vi "Get Border Index.vi"(4 "Y Dimension":i32, 6 "X Dimension":i32, 9 "Min Z":sgl, 11 "Border Vertex Array In":cluster{"X":sgl, "Y":sgl, "Z":sgl}[](array[cluster])) -> (1 "Polygens Index Array":u32[](array[numeric]), 2 "Wireframe Index Array":u32[](array[numeric]), 3 "Border Vertex Array Out":cluster{"X":sgl, "Y":sgl, "Z":sgl}[](array[cluster]))   [LabVIEW 2017, in "3D Mesh.lvclass"]
uses:
  <vilib>/Math Plots/3D Math Plots/3D Mesh/3D Mesh/3D Mesh.lvclass
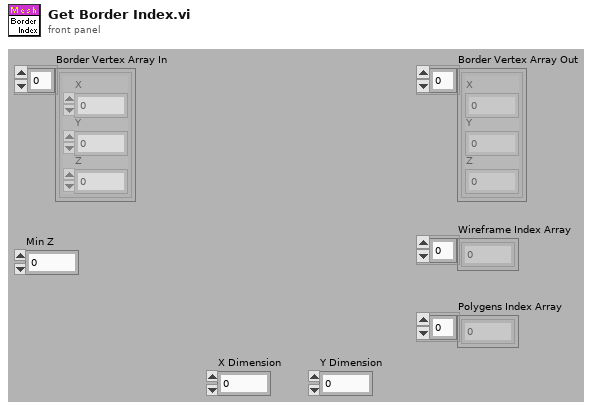
[diagram p1: front panel]
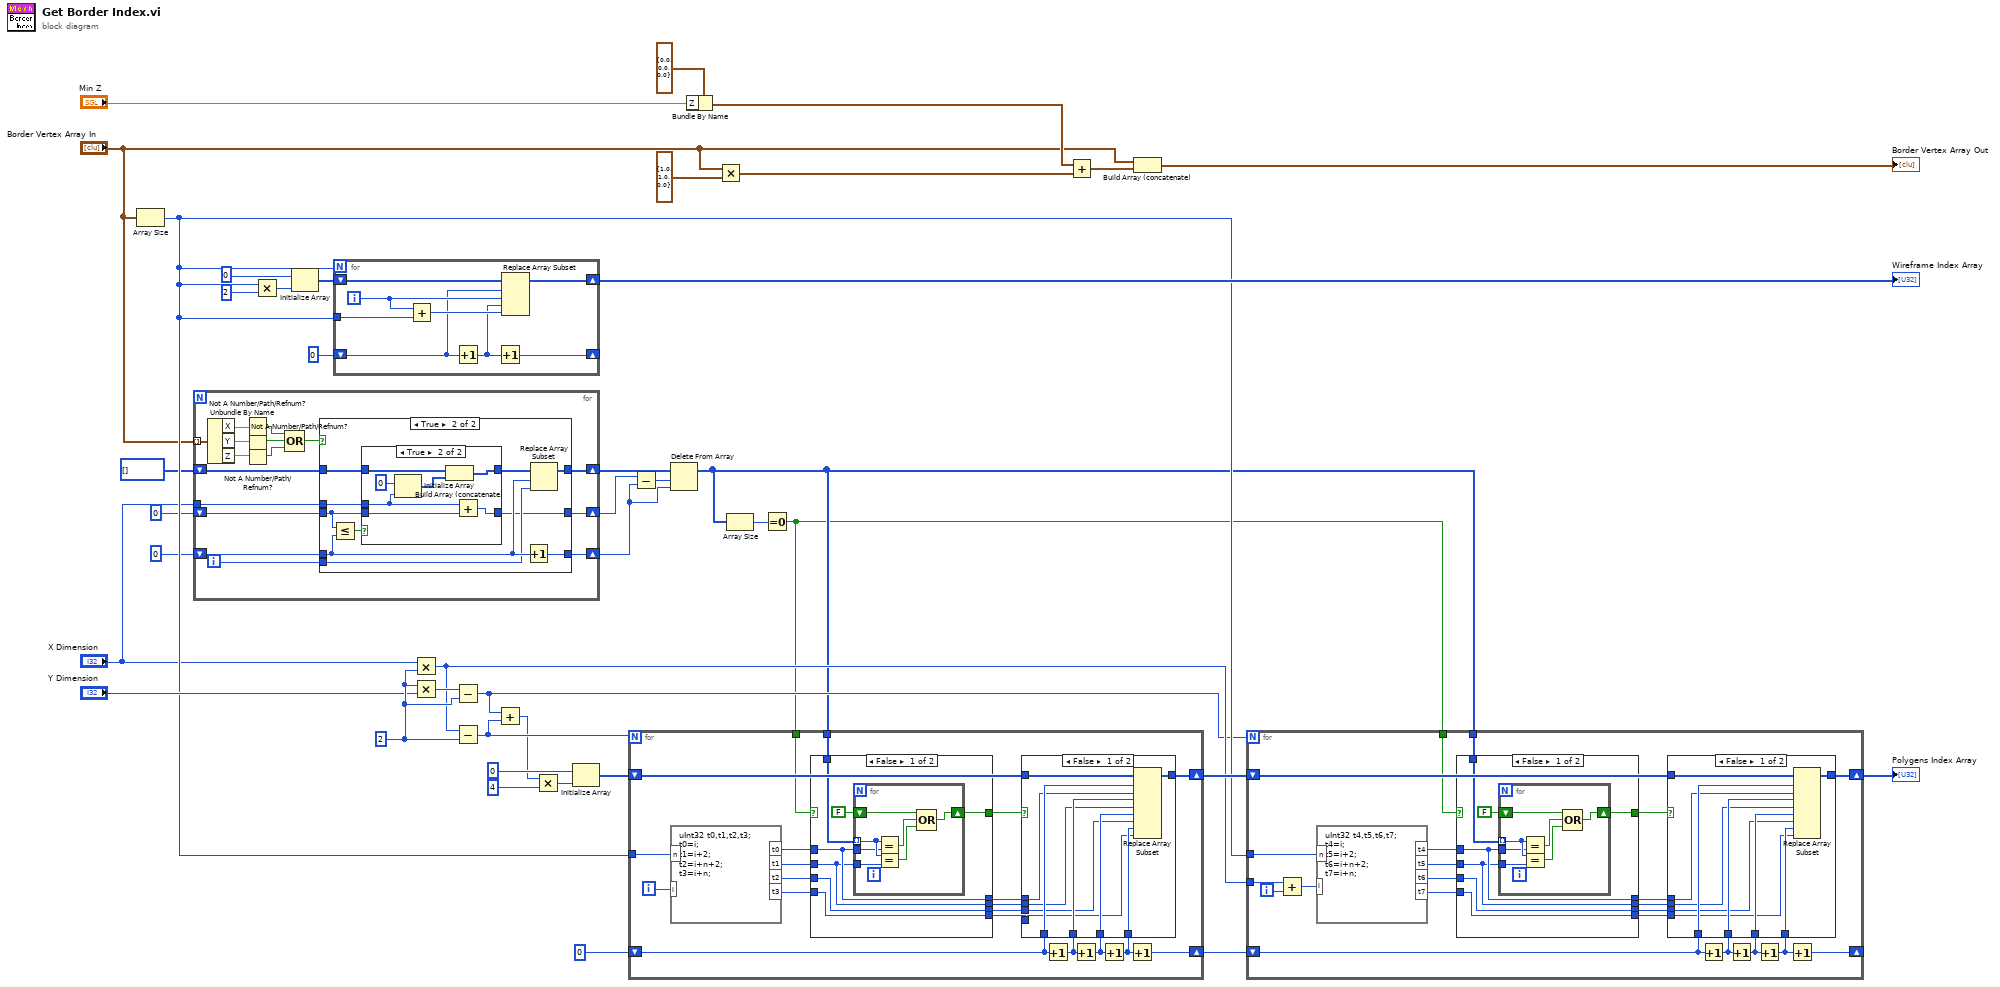
[diagram p0: block diagram]
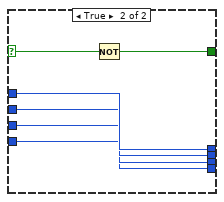
[diagram p5: hidden frame]
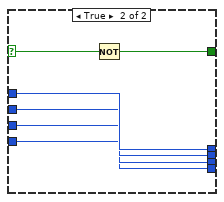
[diagram p7: hidden frame]
diagram:
  w33 = 2 ("y")
  n1 = Array Size(array="Border Vertex Array In") -> (size(s)=w24:i32)
  n2 = for {
    tunnel: "Border Vertex Array In" -> [w57] mode=indexing
    shift-right: [w46] -> w5
    shift-left: 0 -> [w43]
    shift-right: [w47] -> w4
    shift-left: 0 -> [w44]
    shift-right: [w48] -> w6
    shift-left: u32[] [] -> [w45]
    tunnel: "X Dimension" -> [w42]
    i -> [w49]
    n3 = Unbundle By Name(w57) -> ("X"=w56:sgl, "Y"=w55:sgl, "Z"=w54:sgl)
    n4 = Not A Number/Path/Refnum?(number/path/refnum=w56) -> (NaN/Path/Refnum?=w53:bool)
    n5 = Not A Number/Path/Refnum?(number/path/refnum=w55) -> (NaN/Path/Refnum?=w52:bool)
    n6 = Not A Number/Path/Refnum?(number/path/refnum=w54) -> (NaN/Path/Refnum?=w51:bool)
    n7 = Compound Arithmetic op=OR(w53, w52, w51) -> (w50:bool)
    n8 = case shown="True" w50 {
      tunnel: w45 -> [w60 w68]
      tunnel: [w60 w64] -> w48
      tunnel: w49 -> [_ w65]
      tunnel: w43 -> [w59 w66]
      tunnel: [w59 w70] -> w46
      tunnel: w44 -> [w58 w62]
      tunnel: [w58 w63] -> w47
      tunnel: w42 -> [_ w61]
      frame False {
      }
      frame True {
        n9 = Less Or Equal?(x=w62, y=w66) -> (x <= y?=w69:bool)
        n10 = case shown="True" w69 {
          tunnel: w68 -> [w72 w79]
          tunnel: [w72 w78] -> w67
          tunnel: [w71 w74] -> w63
          tunnel: w62 -> [w71 w75]
          tunnel: w61 -> [_ w73]
          frame False {
          }
          frame True {
            n11 = Initialize Array(u32 0, w73) -> (w76:u32[])
            n12 = Build Array (concatenate)(w79, w76) -> (w78:u32[])
            n13 = Add(x=w73, y=w75) -> (x+y=w74:i32)
          }
        }
        n14 = Increment(x=w66) -> (x+1=w70:i32)
        n15 = Replace Array Subset(array=w67, new element=w65, index=w66) -> (w64:u32[])
      }
    }
  }
  n16 = Multiply(x=w24, y=2) -> (x*y=w25:i32)
  n17 = Initialize Array(u32 0, w25) -> (w26:u32[])
  n18 = for {
    N: w24 -> [_]
    shift-right: [w86] -> w39
    shift-left: w26 -> [w87]
    tunnel: w24 -> [w85]
    shift-right: [w82] -> _
    shift-left: 0 ("y") -> [w81]
    i -> [w83]
    n19 = Add(x=w83, y=w85) -> (x+y=w84:i32)
    n20 = Increment(x=w81) -> (x+1=w80:i32)
    n21 = Increment(x=w80) -> (x+1=w82:i32)
    n22 = Replace Array Subset(array=w87, new element #1=w83, index #1=w81, new element #2=w84, index #2=w80) -> (w86:u32[])
  }
  "Wireframe Index Array" <- w39
  n23 = Multiply(x="X Dimension", y=w33) -> (x*y=w32:i32)
  n24 = Multiply(x=w33, y="Y Dimension") -> (x*y=w34:i32)
  n25 = Subtract(x=w34, y=w33) -> (x-y=w18:i32)
  n26 = Subtract(x=w32, y=w33) -> (x-y=w17:i32)
  n27 = Add(x=w18, y=w17) -> (x+y=w16:i32)
  n28 = Multiply(x=w16, y=4) -> (x*y=w20:i32)
  n29 = Initialize Array(u32 0, w20) -> (w15:u32[])
  n30 = Subtract(x=w4, y=w5) -> (x-y=w7:i32)
  n31 = Delete From Array(array=w6, length=w7, index=w5) -> (array with subset deleted=w2:u32[])  [unwired: 1 out]
  n32 = Bundle By Name(cluster=cluster{"X":sgl, "Y":sgl, "Z":sgl} {"X"=0.0, "Y"=0.0, "Z"=0.0} ("3D Point 2"), "Z"="Min Z") -> (w37:cluster{"X":sgl, "Y":sgl, "Z":sgl})
  n33 = Multiply(x="Border Vertex Array In", y=cluster{"X":sgl, "Y":sgl, "Z":sgl} {"X"=1.0, "Y"=1.0, "Z"=0.0} ("3D Point 2")) -> (x*y=w38:cluster{"X":sgl, "Y":sgl, "Z":sgl}[])
  n34 = Array Size(array=w2) -> (size(s)=w3:i32)
  n35 = Equal To 0?(x=w3) -> (x = 0?=w1:bool)
  n36 = for {
    N: w17 -> [_]
    shift-right: [w106] -> w35
    shift-left: w15 -> [w107]
    tunnel: w24 -> [w105]
    shift-right: [w103] -> w13
    shift-left: 0 ("y") -> [w102]
    tunnel: w1 -> [w98]
    tunnel: w2 -> [w97]
    i -> [w104]
    n37 = formula code="uInt32 t0,t1,t2,t3;\nt0=i;\nt1=i+2;\nt2=i+n+2;\nt3=i+n;"("n"=w105, "i"=w104) -> ("t0"=w96:u32, "t1"=w95:u32, "t2"=w94:u32, "t3"=w93:u32)
    n38 = case shown="False" w98 {
      selector: w98 -> [_ w134]
      tunnel: [w122 w138] -> w92
      tunnel: w96 -> [w122 w138]
      tunnel: [w121 w137] -> w91
      tunnel: w95 -> [w121 w137]
      tunnel: [w120 w136] -> w90
      tunnel: w94 -> [w120 w136]
      tunnel: [w119 w135] -> w89
      tunnel: w93 -> [w119 w135]
      tunnel: w97 -> [w125 _]
      tunnel: [w123 w133] -> w88
      frame False {
        n39 = for {
          tunnel: w125 -> [w132] mode=indexing
          tunnel: w122 -> [w131]
          tunnel: w121 -> [w126]
          shift-right: [w128] -> w123
          shift-left: FALSE -> [w127]
          n40 = Equal?(x=w132, y=w131) -> (x = y?=w130:bool)
          n41 = Equal?(x=w132, y=w126) -> (x = y?=w129:bool)
          n42 = Compound Arithmetic op=OR(w127, w130, w129) -> (w128:bool)
        }
      }
      frame True {
        n43 = Not(x=w134) -> (.not. x?=w133:bool)
      }
    }
    n44 = Increment(x=w102) -> (x+1=w101:i32)
    n45 = Increment(x=w101) -> (x+1=w100:i32)
    n46 = Increment(x=w100) -> (x+1=w99:i32)
    n47 = case shown="False" w88 {
      tunnel: w107 -> [w117 w118]
      tunnel: [w116 w118] -> w106
      tunnel: w102 -> [w115 _]
      tunnel: w101 -> [w114 _]
      tunnel: w100 -> [w113 _]
      tunnel: w99 -> [w112 _]
      tunnel: w92 -> [w111 _]
      tunnel: w91 -> [w110 _]
      tunnel: w90 -> [w109 _]
      tunnel: w89 -> [w108 _]
      frame False {
        n48 = Replace Array Subset(array=w117, new element #1=w111, index #1=w115, new element #2=w110, index #2=w114, new element #3=w109, index #3=w113, new element #4=w108, index #4=w112) -> (w116:u32[])
      }
      frame True {
      }
    }
    n49 = Increment(x=w99) -> (x+1=w103:i32)
  }
  n50 = Add(x=w37, y=w38) -> (x+y=w36:cluster{"X":sgl, "Y":sgl, "Z":sgl}[])
  n51 = Build Array (concatenate)("Border Vertex Array In", w36) -> (→"Border Vertex Array Out":cluster{"X":sgl, "Y":sgl, "Z":sgl}[])
  n52 = for {
    N: w18 -> [_]
    shift-right: [w155] -> w31
    shift-left: w35 -> [w156]
    tunnel: w24 -> [w160]
    tunnel: w32 -> [w159]
    shift-right: [w154] -> _
    shift-left: w13 -> [w153]
    tunnel: w2 -> [w149]
    tunnel: w1 -> [w148]
    i -> [w158]
    n53 = Add(x=w159, y=w158) -> (x+y=w157:i32)
    n54 = formula code="uInt32 t4,t5,t6,t7;\nt4=i;\nt5=i+2;\nt6=i+n+2;\nt7=i+n;"("n"=w160, "i"=w157) -> ("t4"=w147:u32, "t5"=w146:u32, "t6"=w145:u32, "t7"=w144:u32)
    n55 = case shown="False" w148 {
      selector: w148 -> [_ w187]
      tunnel: [w175 w191] -> w143
      tunnel: w147 -> [w175 w191]
      tunnel: [w174 w190] -> w142
      tunnel: w146 -> [w174 w190]
      tunnel: [w173 w189] -> w141
      tunnel: w145 -> [w173 w189]
      tunnel: [w172 w188] -> w140
      tunnel: w144 -> [w172 w188]
      tunnel: w149 -> [w178 _]
      tunnel: [w176 w186] -> w139
      frame False {
        n56 = for {
          tunnel: w178 -> [w185] mode=indexing
          tunnel: w175 -> [w184]
          tunnel: w174 -> [w179]
          shift-right: [w181] -> w176
          shift-left: FALSE -> [w180]
          n57 = Equal?(x=w185, y=w184) -> (x = y?=w183:bool)
          n58 = Equal?(x=w185, y=w179) -> (x = y?=w182:bool)
          n59 = Compound Arithmetic op=OR(w180, w183, w182) -> (w181:bool)
        }
      }
      frame True {
        n60 = Not(x=w187) -> (.not. x?=w186:bool)
      }
    }
    n61 = Increment(x=w153) -> (x+1=w152:i32)
    n62 = Increment(x=w152) -> (x+1=w151:i32)
    n63 = Increment(x=w151) -> (x+1=w150:i32)
    n64 = case shown="False" w139 {
      tunnel: w156 -> [w170 w171]
      tunnel: [w169 w171] -> w155
      tunnel: w153 -> [w168 _]
      tunnel: w152 -> [w167 _]
      tunnel: w151 -> [w166 _]
      tunnel: w150 -> [w165 _]
      tunnel: w143 -> [w164 _]
      tunnel: w142 -> [w163 _]
      tunnel: w141 -> [w162 _]
      tunnel: w140 -> [w161 _]
      frame False {
        n65 = Replace Array Subset(array=w170, new element #1=w164, index #1=w168, new element #2=w163, index #2=w167, new element #3=w162, index #3=w166, new element #4=w161, index #4=w165) -> (w169:u32[])
      }
      frame True {
      }
    }
    n66 = Increment(x=w150) -> (x+1=w154:i32)
  }
  "Polygens Index Array" <- w31
